vi "Update Saving Status.vi"(8 "error in":errorcluster, 11 "File Actor in":refnum<class "File Actor.lvclass">) -> (0 "error out":errorcluster, 3 "File Actor out":refnum<class "File Actor.lvclass">)   [LabVIEW 2017, in "File Library.lvlib" / "File Actor.lvclass"]
doc: "This method of the File Actor object is used to tell the caller what the current file status is. This status generally will not differe from that directed by the caller, but in some cases, such as at configuration or if there is an error, the status may differ from that of the caller. \n\nThis VI is in community scope so it may be used by the Exe Write object to update when writing."
uses:
  File Actor.lvclass
  C:/Program Files (x86)/National Instruments/LabVIEW 2017/vi.lib/ActorFramework/Actor/Actor.lvclass
  File Actor.lvclass/File Actor.ctl
  <vilib>/ActorFramework/Actor/Actor.lvclass/Actor.ctl
  Messages/Abstract/Saving File Message/Saving File Message.lvclass/Saving File Message.ctl
  <vilib>/ActorFramework/Message Enqueuer/Message Enqueuer.lvclass/Message Enqueuer.ctl
  Messages/Abstract/Saving File Message/Write Saving.vi
  Messages/Abstract/Saving File Message/Saving File Message.lvclass
  C:/Program Files (x86)/National Instruments/LabVIEW 2017/vi.lib/ActorFramework/Message/Message.lvclass
  <vilib>/ActorFramework/Message Priority Queue/Priority Enqueue.vi
  <vilib>/ActorFramework/Actor/Actor.lvclass
  <vilib>/ActorFramework/Message Enqueuer/Message Enqueuer.lvclass
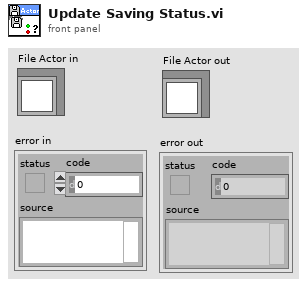
[diagram p1: front panel]
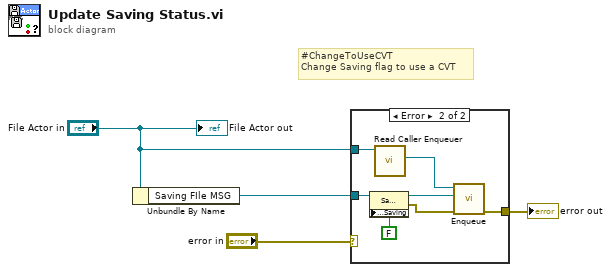
[diagram p0: block diagram]
diagram:
  # "#ChangeToUseCVT\nChange Saving flag to use a CVT"
  n1 = Unbundle By Name("File Actor in") -> ("Saving FIle MSG"=w2:refnum<class "Saving File Message.lvclass">)
  n2 = case shown="Error" "error in" {
    tunnel: [_ w9] -> w4
    tunnel: "File Actor in" -> [_ w8]
    tunnel: w2 -> [_ w7]
    frame No Error {
    }
    frame Error {
      n3 = property class="Saving Main File MSG"(reference=w7, "Accessors:Saving"=FALSE ("t")) -> (reference out=w11:refnum<class "Saving File Message.lvclass">, error out=w6:errorcluster)  [unwired: 1 in]
      n4 = call <vilib>:"Read Caller Enqueuer.vi"("Actor"=w8) -> ("Caller Enqueuer"=w10:refnum<class "Message Enqueuer.lvclass">)  [unwired: 10 in]
      n5 = call <vilib>:"Enqueue.vi"("error in (no error)"=w6, "Message"=w11, "Message Enqueuer in"=w10) -> ("error out"=w9:errorcluster)  [unwired: 7 in, 1 out]
    }
  }
  "error out" <- w4
  "File Actor out" <- "File Actor in"
